vi "BML_Write_Only_Opcode.vi"() -> ()   [LabVIEW 2016]
uses:
  Classes/Config_Read/Config_Read_BML.lvclass
  Classes/BML_DigiPattern_Generator/DigiPattern_Generator.lvclass
  Classes/BML_Frame_Write_Opcode/BML_Frame_Write_Opcode.lvclass
  C:/Users/8135/Desktop/BML_Pattern_Gen/BeamLink_Pattern_Gen/BML_Pattern_Gen_Refactor/Classes/BML_Frame_Root/BML_Frame_Root.lvclass
  Classes/BML_Frame_RW/BML_Frame_RW.lvclass
  Classes/BML_Frame_SetID/BML_Frame_SetID.lvclass
  Classes/Config_Read/RW_Option.ctl
  Classes/Config_Read/BurstLength.ctl
  Classes/Config_Read/OperationMode.ctl
  Classes/Config_Read/Frame_Data.ctl
panel:
  out "error out":errorcluster
  in  "PinMap":path
  in  "ChipID":u8=1
  in  "Config Path":path
  in  "error in (no error)":errorcluster
  # "OPCODE supported here. WR frame only"
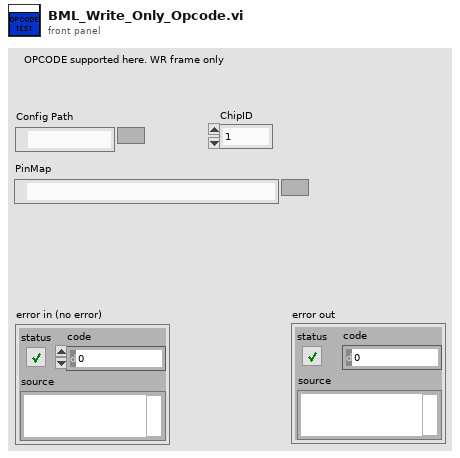
[diagram p1: front panel]
types:
  T1 = typedef "Config_Read_BML.lvclass/Frame_Data.ctl" = cluster{"Pattern_Name":string, "Operation Mode":T2, "BurstLength":T3, "FSN":u8, "Start_Addr":u16, "Data":u8[], "R/W?":T4, "Opcode":string[]}
  T2 = typedef "Config_Read_BML.lvclass/OperationMode.ctl" = enum8{"Normal", "ImmeEffect", "InitSlaveID", "LoadData"}
  T3 = typedef "Config_Read_BML.lvclass/BurstLength.ctl" = enum8{"0", "2", "3", "4", "5", "8", "16", "32"}
  T4 = typedef "Config_Read_BML.lvclass/RW_Option.ctl" = enum16{"Read", "Write", "R/W"}
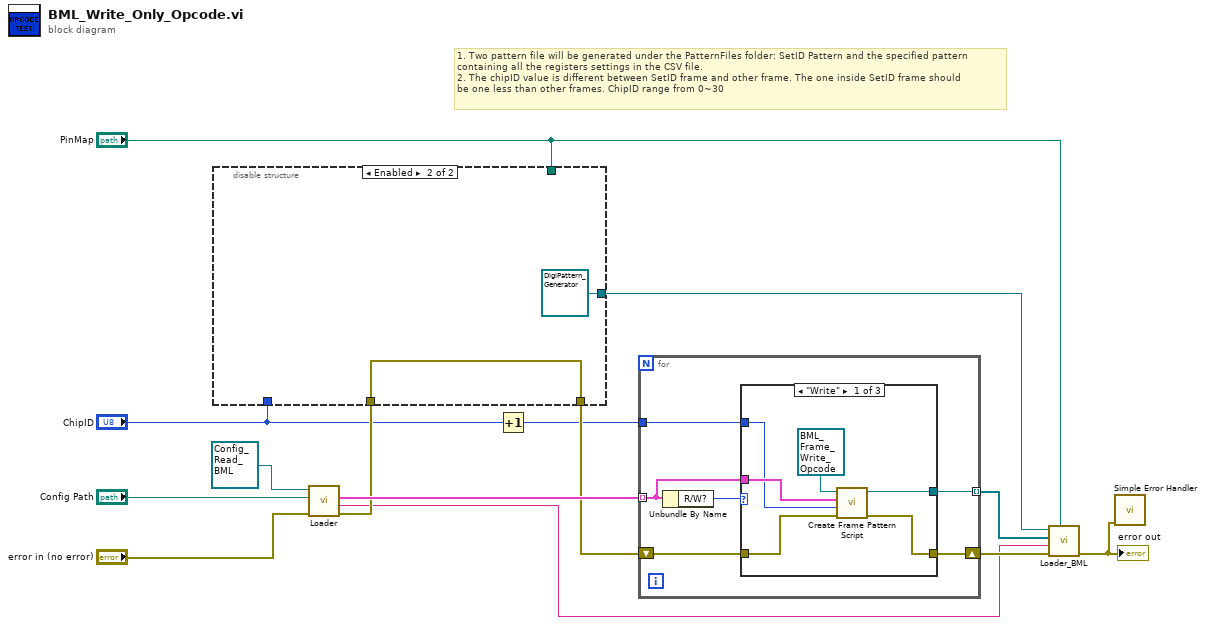
[diagram p0: block diagram]
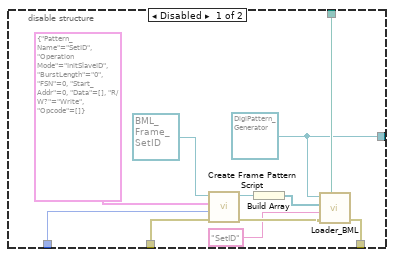
[diagram p2: hidden frame]
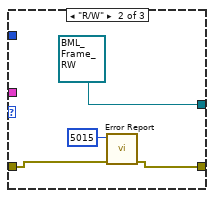
[diagram p3: hidden frame]
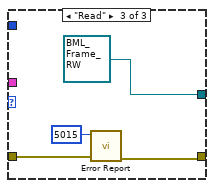
[diagram p4: hidden frame]
diagram:
  # "1. Two pattern file will be generated under the PatternFiles folder: SetID Pattern and the specified pattern\ncontaining all the registers settings in the CSV file.\n2. The chipID value is different between SetID frame and other frame. The one inside SetID frame should \nbe one less than other frames. ChipID range from 0~30"
  n1 = call "Loader.vi"("error in (no error)"="error in (no error)", "Path"="Config Path", "Config_Read.lvclass"=refnum<class "Config_Read_BML.lvclass"> refnum) -> ("error out"=w10:errorcluster, "Pattern_Name"=w3:string, "FRM_Data_Array"=w11:T1[])  [unwired: 5 in, 1 out]
  n2 = disable-structure shown="Enabled" {
    disable-tunnel: w10 -> [w23 w26]
    disable-tunnel: [w22 w26] -> w9
    disable-tunnel: "ChipID" -> [w19 _]
    disable-tunnel: "PinMap" -> [w16 _]
    disable-tunnel: [w15 refnum<class "DigiPattern_Generator.lvclass"> refnum ("BML_DigiPattern_Generator.lvclass")] -> w2
    frame Disabled {
      w15 = refnum<class "DigiPattern_Generator.lvclass"> refnum ("BML_DigiPattern_Generator.lvclass")
      n3 = call-dynamic "Create Frame Pattern Script.vi"("error in (no error)"=w23, "ChipID"=w19, "Frame_Data"=T1 {"Pattern_Name"="SetID", "Operation Mode"=enum."InitSlaveID", "BurstLength"=enum."0", "FSN"=0, "Start_Addr"=0, "Data"=[], "R/W?"=enum."Write", "Opcode"=[]}, "BML_Frame_SetID in"=refnum<class "BML_Frame_SetID.lvclass"> refnum ("BML_Frame_SetID.lvclass")) -> ("error out"=w21:errorcluster, "BML_Frame_SetID out"=w18:refnum<class "BML_Frame_SetID.lvclass">)  [unwired: 6 in]
      n4 = Build Array(w18) -> (w17:refnum<class "BML_Frame_SetID.lvclass">[])
      n5 = call "Loader_BML.vi"("PinMap"=w16, "error in (no error)"=w21, "Pattern Name"="SetID", "BML Frame Array"=w17, "BML_DigiPattern_Generator.lvclass"=w15) -> ("error out"=w22:errorcluster)  [unwired: 5 in, 1 out]
    }
    frame Enabled {
    }
  }
  n6 = Increment(x="ChipID") -> (x+1=w7:u8)
  n7 = for {
    tunnel: w11 -> [w31] mode=indexing
    tunnel: w7 -> [w30]
    shift-right: [w29] -> w6
    shift-left: w9 -> [w32]
    tunnel: [w28] -> w5 mode=indexing
    n8 = Unbundle By Name(w31) -> ("R/W?"=w33:T4)
    n9 = case shown="\"Write\"" w33 {
      tunnel: w32 -> [w38 w42 w44]
      tunnel: w31 -> [w39 _ _]
      tunnel: w30 -> [w37 _ _]
      tunnel: [w36 refnum<class "BML_Frame_RW.lvclass"> refnum ("BML_Frame_RW.lvclass") refnum<class "BML_Frame_RW.lvclass"> refnum ("BML_Frame_RW.lvclass")] -> w28
      tunnel: [w35 w41 w45] -> w29
      frame "Write" {
        n10 = call-dynamic "Create Frame Pattern Script.vi"("error in (no error)"=w38, "ChipID"=w37, "Frame_Data"=w39, "BML_Frame_Write_Opcode in"=refnum<class "BML_Frame_Write_Opcode.lvclass"> refnum ("BML_Frame_Write_Opcode.lvclass")) -> ("error out"=w35:errorcluster, "BML_Frame_Write_Opcode out"=w36:refnum<class "BML_Frame_Write_Opcode.lvclass">)  [unwired: 6 in]
      }
      frame "R/W" {
        n11 = call "Error Report.vi"("error in (no error)"=w42, "Error Code"=i16 5015) -> ("error out"=w41:errorcluster)  [unwired: 9 in]
      }
      frame "Read" {
        n12 = call "Error Report.vi"("error in (no error)"=w44, "Error Code"=i16 5015) -> ("error out"=w45:errorcluster)  [unwired: 9 in]
      }
    }
  }
  n13 = call "Loader_BML.vi"("PinMap"="PinMap", "error in (no error)"=w6, "Pattern Name"=w3, "BML Frame Array"=w5, "BML_DigiPattern_Generator.lvclass"=w2) -> ("error out"=w1:errorcluster)  [unwired: 5 in, 1 out]
  "error out" <- w1
  n14 = call <vilib>:"Simple Error Handler.vi"("error in (no error)"=w1) -> ()  [unwired: 4 in, 5 out]
